vi "未命名 1.vi"() -> ()   [LabVIEW 2019]
uses:
  lib/Lake Shore 335/Lake Shore 335.lvlib
  <vilib>/Modbus/master/Modbus Master.lvclass
panel:
  in  "Heater Output (1:1)":u16(ring)=1 items=["1"=1, "2"=2]
  in  "Input (0:A)":u16(ring) items=["A", "B"]
  out "Staus":u16(ring) items=["Unknow", "Stable", "Following", "Unfollowing"]
  out "Temp":dbl format="%.4f"
  out "Setpoint":dbl format="%.4f"
  out "Ramping Active":bool
  out "Heater Range":u16(ring) items=["Off", "Low (On)", "Medium", "High"]
  out "Output Value":dbl format="%.1f"
  out "压缩机远程开启":bool
  out "压缩机开启":bool
  out "error out 3":errorcluster
  in  "压缩机自动停止":bool
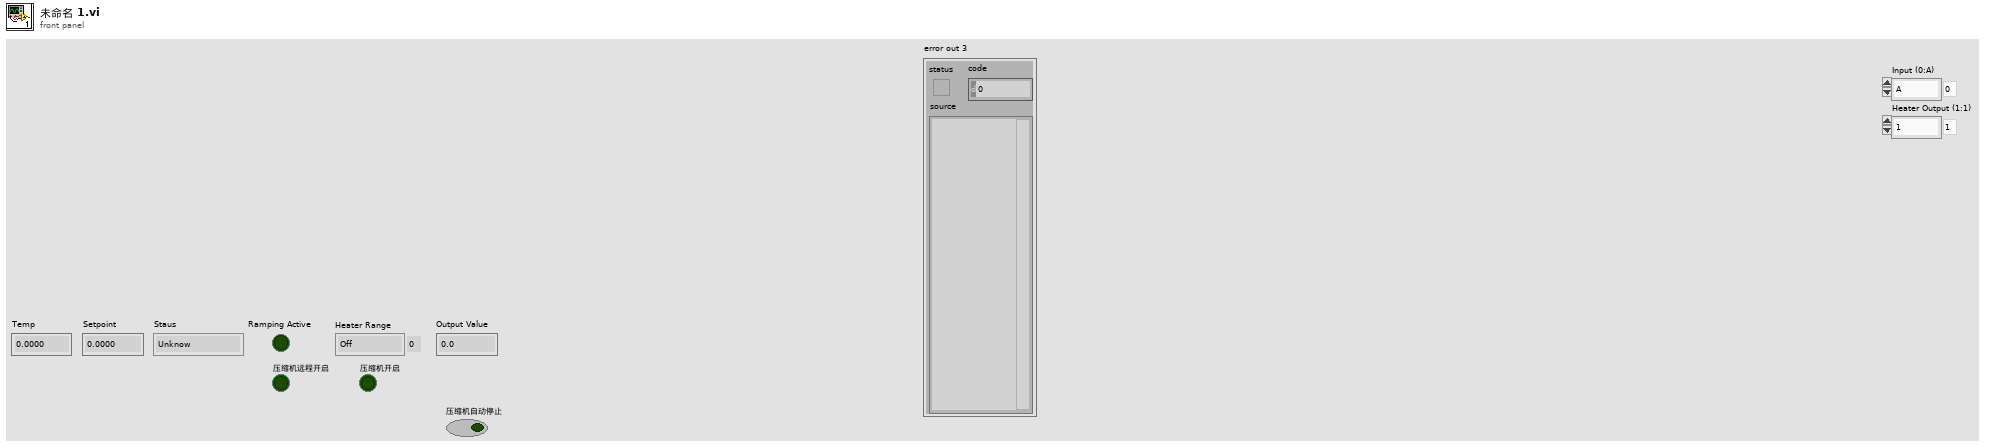
[diagram p1: front panel]
types:
  T1 = typedef "Semaphore RefNum" = refnum<k1>
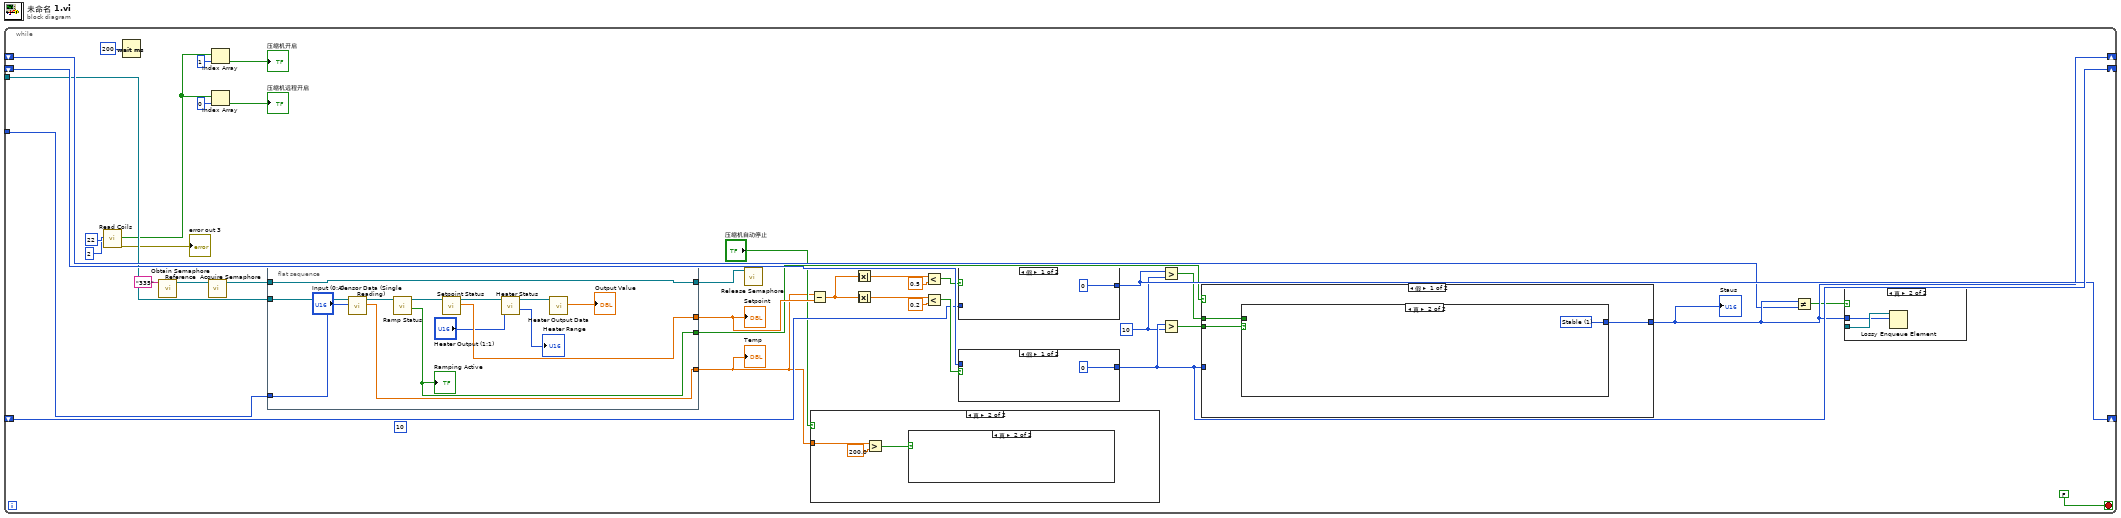
[diagram p0: block diagram]
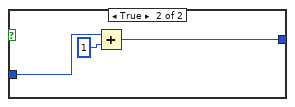
[diagram p5: hidden frame]
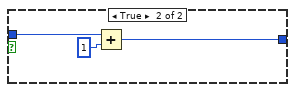
[diagram p6: hidden frame]
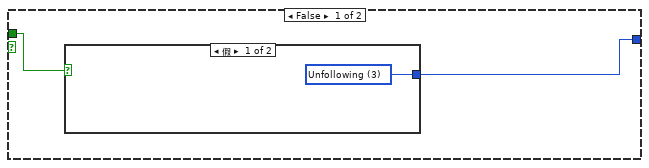
[diagram p7: hidden frame]
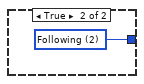
[diagram p8: hidden frame]
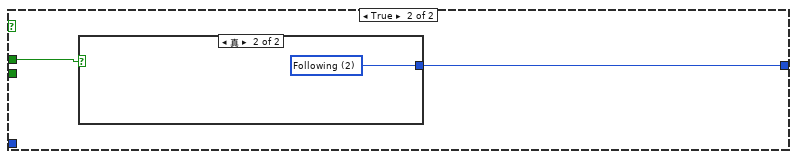
[diagram p9: hidden frame]
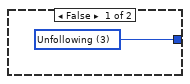
[diagram p10: hidden frame]
diagram:
  n1 = while {
    tunnel: _ -> [w11]
    shift-right: [w27] -> _
    shift-left: _ -> [w34]
    shift-right: [w26] -> _
    shift-left: _ -> [w29]
    tunnel: [w12] -> _
    shift-right: [w22] -> _
    shift-left: _ -> [w21]
    stop <- FALSE stop-if-true
    w25 = 10 ("y")
    (unwired) 10
    n2 = call-dynamic "Read Coils.vi"("number of coils"=u16 2 ("number of inputs"), "starting address"=u16 22) -> ("error out"=→"error out 3":errorcluster, "coil values"=w7:bool[])  [unwired: 7 in, 1 out]
    n3 = Wait (ms)(milliseconds to wait=u32 200) -> ()  [unwired: 1 out]
    n4 = call <vilib>:"Obtain Semaphore Reference.vi"("name (unnamed)"="335") -> ("semaphore"=w17:T1)  [unwired: 4 in, 2 out]
    n5 = call <vilib>:"Acquire Semaphore.vi"("semaphore"=w17) -> ("semaphore out"=w16:T1)  [unwired: 4 in, 2 out]
    n6 = Index Array(array=w7, index=1) -> (element=→"压缩机开启":bool)
    n7 = Index Array(array=w7, index=0) -> (element=→"压缩机远程开启":bool)
    n8 = flat-sequence {
      tunnel: w16 -> [w53]
      tunnel: [w53] -> w15
      tunnel: [w52] -> w14
      tunnel: [w51] -> w13
      tunnel: ["Input (0:A)"] -> w12
      tunnel: w11 -> [w48]
      tunnel: [w42] -> w1
      frame #0 {
        n9 = call "Sensor Data (Single Reading).vi"("Input (0:A)"="Input (0:A)", "VISA resource name"=w48) -> ("Sensor Data"=w42:dbl, "VISA resource name out"=w47:refnum<visa-resource-name>)  [unwired: 7 in, 1 out]
        n10 = call "Ramp Status.vi"("VISA resource name"=w47) -> ("Ramping Active"=w51:bool, "VISA resource name out"=w50:refnum<visa-resource-name>)  [unwired: 6 in, 3 out]
        "Ramping Active" <- w51
        n11 = call "Setpoint Status.vi"("VISA resource name"=w50) -> ("Setpoint"=w52:dbl, "VISA resource name out"=w46:refnum<visa-resource-name>)  [unwired: 8 in, 1 out]
        n12 = call "Heater Status.vi"("Heater Output (1:1)"="Heater Output (1:1)", "VISA resource name"=w46) -> ("Heater Range"=→"Heater Range":u16, "VISA resource name out"=w44:refnum<visa-resource-name>)  [unwired: 5 in, 3 out]
        n13 = call "Heater Output Data.vi"("VISA resource name"=w44) -> ("Output Value"=→"Output Value":dbl)  [unwired: 8 in, 2 out]
      }
    }
    n14 = call <vilib>:"Release Semaphore.vi"("semaphore"=w15) -> ()  [unwired: 5 in, 2 out]
    n15 = case shown="真" "压缩机自动停止" {
      tunnel: w1 -> [_ w40]
      frame False {
      }
      frame True {
        n16 = Greater?(x=w40, y=200.0) -> (0:w38:bool)
        n17 = case shown="真" w38 {
          frame False {
          }
          frame True {
          }
        }
      }
    }
    n18 = Subtract(x=w1, y=w14) -> (x-y=w31:dbl)
    n19 = Absolute Value(x=w31) -> (abs(x)=w33:dbl)
    n20 = Absolute Value(x=w31) -> (abs(x)=w35:dbl)
    n21 = Less?(x=w33, y=0.5) -> (x < y?=w30:bool)
    n22 = Less?(x=w35, y=0.2) -> (x < y?=w36:bool)
    n23 = case shown="假" w30 {
      tunnel: w29 -> [_ w59]
      tunnel: [0 w57] -> w26
      frame False {
      }
      frame True {
        n24 = Add(x=w59, y=1) -> (x+y=w57:i32)
      }
    }
    n25 = case shown="假" w36 {
      tunnel: w34 -> [_ w63]
      tunnel: [0 w61] -> w27
      frame False {
      }
      frame True {
        n26 = Add(x=w63, y=1) -> (x+y=w61:i32)
      }
    }
    n27 = Greater?(x=w26, y=w25) -> (0:w23:bool)
    n28 = Greater?(x=w27, y=w25) -> (0:w24:bool)
    n29 = case shown="假" w13 {
      tunnel: w27 -> [_ _]
      tunnel: w24 -> [w66 _]
      tunnel: w23 -> [w65 w73]
      tunnel: [w64 w72] -> w22
      frame False {
        n30 = case shown="真" w66 {
          tunnel: [w67 w71] -> w64
          tunnel: w65 -> [w68 _]
          frame False {
            n31 = case shown="假" w68 {
              tunnel: [w69 w70] -> w67
              frame False {
                w69 = u16 3 items=["Unknow", "Stable", "Following", "Unfollowing"]
              }
              frame True {
                w70 = u16 2 items=["Unknow", "Stable", "Following", "Unfollowing"]
              }
            }
          }
          frame True {
            w71 = u16 1 items=["Unknow", "Stable", "Following", "Unfollowing"]
          }
        }
      }
      frame True {
        n32 = case shown="真" w73 {
          tunnel: [w74 w75] -> w72
          frame False {
            w74 = u16 3 items=["Unknow", "Stable", "Following", "Unfollowing"]
          }
          frame True {
            w75 = u16 2 items=["Unknow", "Stable", "Following", "Unfollowing"]
          }
        }
      }
    }
    "Staus" <- w22
    n33 = Not Equal?(x=w22, y=w21) -> (x != y?=w20:bool)
    n34 = case shown="真" w20 {
      tunnel: _ -> [_ w55]
      tunnel: w22 -> [_ w54]
      frame False {
      }
      frame True {
        n35 = Lossy Enqueue Element(queue=w55, element=w54) -> ()  [unwired: 1 in, 4 out]
      }
    }
    "Temp" <- w1
    "Setpoint" <- w14
  }
